vi "Daten Serialisieren - Messwerte.vi"(9 "Frame-ID":u32, 10 "Aktuelle Zeit":timestamp, 11 "Messdaten":sgl[](array[numeric])) -> (2 "data":T1[](array[typedef])=[{"timestamp"=timestamp(0 s since 1904-01-01), "payload"=[0, 2, 3, 4, 5, 6, 7, 8], "identifier"=2, "type"=0, "extended?"=FALSE, "echo?"=FALSE}, {"timestamp"=timestamp(0 s since 1904-01-01), "payload"=[0, 1, 2, 3, 4, 5, 6, 7], "identifier"=3, "type"=0, "extended?"=FALSE, "echo?"=FALSE}] {"payload" format="%x"; "timestamp" format="%<%.7X\n%x>T"; "type" items=["CAN Data"=0, "CAN Remote"=1, "CAN Bus Error"=2, "CAN 2.0 Data"=8, "CAN FD Data"=16, "CAN FD+BRS Data"=24, "J1939 Data"=192, "Delay"=224, "Log Trigger"=225, "Start Trigger"=226]; "identifier" format="%x"})   [LabVIEW 2020, in "CAN Interface.lvlib"]
uses:
  195161_2023-03-15/cRIO/CAN Interface/CAN Interface.lvlib
  <vilib>/xnet/xnet.llb/XNET Frame Type CAN.ctl
  <vilib>/xnet/xnet.llb/XNET Frame CAN.ctl
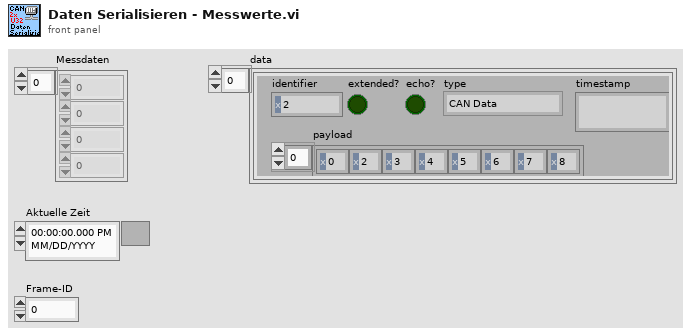
[diagram p1: front panel]
types:
  T1 = typedef "XNET Frame CAN.ctl" = cluster{"timestamp":timestamp, "payload":u8[], "identifier":u32, "type":T2, "extended?":bool, "echo?":bool}
  T2 = typedef "XNET Frame Type CAN.ctl" = u8
  T3 = enum16{"big-endian, network order", "native, host order", "little-endian"}
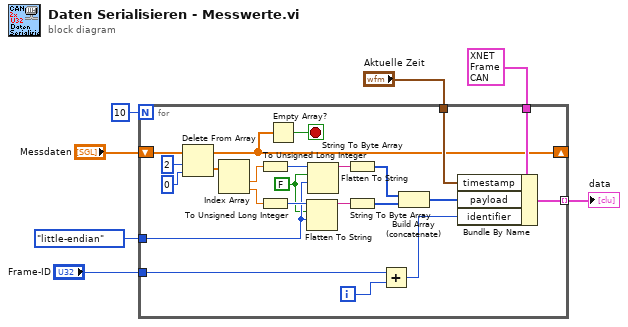
[diagram p0: block diagram]
diagram:
  n1 = for {
    N: 10 -> [_]
    tunnel: T3."little-endian" ("Byte-Reihenfolge (0:Big-Endian, Netzwerkreihenfolge)") -> [w11]
    tunnel: T1 {"timestamp"=timestamp(0 s since 1904-01-01), "payload"=[0, 2, 3, 4, 5, 6, 7, 8], "identifier"=2, "type"=0, "extended?"=FALSE, "echo?"=FALSE} ("CAN frame") -> [w29]
    tunnel: "Frame-ID" -> [w27]
    tunnel: "Aktuelle Zeit" -> [w25]
    tunnel: [w24] -> w3 mode=indexing
    shift-right: [w13] -> _
    shift-left: "Messdaten" -> [w22]
    i -> [w28]
    stop <- w12 stop-if-true
    w10 = FALSE ("Array- oder String-Größe voranstellen? (T)")
    n2 = Delete From Array(array=w22, length=2 ("Länge"), index=0 ("Index")) -> (deleted portion=w19:sgl[], array with subset deleted=w13:sgl[])
    n3 = Index Array(array=w19) -> (element #1=w9:sgl, element #2=w8:sgl)  [unwired: 2 in]
    n4 = To Unsigned Long Integer(number=w9) -> (unsigned 32bit integer=w18:u32)
    n5 = To Unsigned Long Integer(number=w8) -> (unsigned 32bit integer=w23:u32)
    n6 = Empty Array?(array=w13) -> (empty?=w12:bool)
    n7 = Flatten To String(anything=w23, prepend array or string size? (T)=w10, byte order (0:big-endian, network order)=w11) -> (data string=w30:string)  [unwired: 1 in, 2 out]
    n8 = Flatten To String(anything=w18, prepend array or string size? (T)=w10, byte order (0:big-endian, network order)=w11) -> (data string=w17:string)  [unwired: 1 in, 2 out]
    n9 = String To Byte Array(string=w17) -> (unsigned byte array=w16:u8[])
    n10 = String To Byte Array(string=w30) -> (unsigned byte array=w15:u8[])
    n11 = Add(x=w27, y=w28) -> (x+y=w26:u32)
    n12 = Build Array (concatenate)(w16, w15) -> (w14:u8[])
    n13 = Bundle By Name(cluster=w29, "timestamp"=w25, "payload"=w14, "identifier"=w26) -> (w24:T1)
  }
  "data" <- w3
